vi "Action Name.vi"(11 "CLIAction in":refnum<class "CLIAction.lvclass">) -> (2 "Action Name":string)   [LabVIEW 2020, in "GPackTools.lvlib" / "CLIAction.lvclass"]
uses:
  CLIAction.lvclass
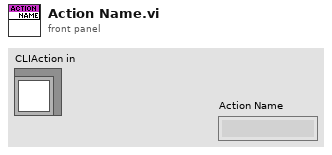
[diagram p1: front panel]
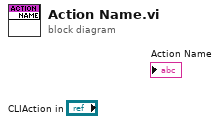
[diagram p0: block diagram]
diagram:
